vi "Create Instrument Addon.vi"(8 "error in (no error)":errorcluster, 9 "CD Config Path (.dat)":path, 10 "Name":string, 11 "Custom Devices Ref":refnum<k24>) -> (0 "error out":errorcluster, 3 "Custom Devices Ref":refnum<k24>)   [LabVIEW 2019, in "Instrument System Definition API.lvlib"]
uses:
  Instrument System Definition API.lvlib
  NationalInstruments.VeriStand.SystemDefinitionAPI
  Addon/Addon Shared/SubVIs/Constants.vi
  Addon/Addon Shared/Instrument Addon Shared.lvlib
  <vilib>/NI/NI VeriStand Custom Device Import and Export Tool/ImportExport.lvlib
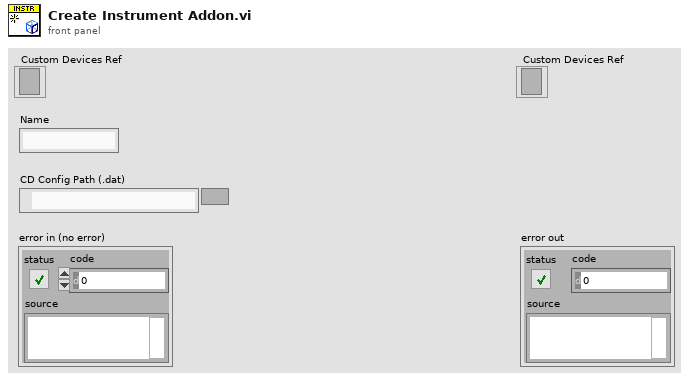
[diagram p1: front panel]
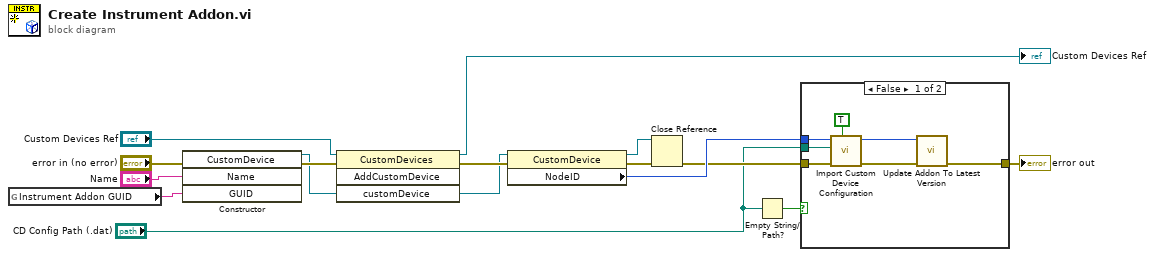
[diagram p0: block diagram]
diagram:
  n1 = global read "Constants.vi" "Instrument Addon GUID"() -> (w14:string)
  n2 = constructor class="CustomDevice"(error in="error in (no error)", "Name"="Name", "GUID"=w14) -> (reference out=w7:refnum<k24>, error out=w9:errorcluster)  [unwired: 2 in, 3 out]
  n3 = invoke class="CustomDevices" method="AddCustomDevice"(reference="Custom Devices Ref", error in=w9, "customDevice"=w7) -> (reference out=→"Custom Devices Ref":refnum<k24>, error out=w8:errorcluster)  [unwired: 1 in, 2 out]
  n4 = property class="CustomDevice"(reference=w7, error in=w8) -> (reference out=w5:refnum<k24>, error out=w4:errorcluster, "NodeID"=w12:u64)
  n5 = Close Reference(reference=w5, error in (no error)=w4) -> (error out=w3:errorcluster)
  n6 = Empty String/Path?(string/path="CD Config Path (.dat)") -> (empty?=w1:bool)
  n7 = case shown="False" w1 {
    tunnel: w12 -> [w22 _]
    tunnel: [w17 w23] -> w11
    tunnel: w3 -> [w20 w23]
    tunnel: "CD Config Path (.dat)" -> [w19 _]
    frame False {
      n8 = call <vilib>:"Import Custom Device Configuration.vi"("Overwrite Existing?"=TRUE, "error in (no error)"=w20, "Path"=w19, "NodeID"=w22) -> ("error out"=w18:errorcluster, "NodeID out"=w16:u64)  [unwired: 5 in, 1 out]
      n9 = call "Update Addon To Latest Version.vi"("error in (no error)"=w18, "Device Item Ref in"=w16) -> ("error out"=w17:errorcluster)  [unwired: 8 in, 1 out]
    }
    frame True {
    }
  }
  "error out" <- w11
